vi "Insert_Event_Log(Error_glue).vi"(8 "data":string="790", 9 "message":string="B", 10 "id":string="NG", 11 "DBlink":string="Driver={ODBC Driver 17 for SQL Server};Server=localhost\\SQLEXPRESS;Database=ZDX201;UID=labview;PWD=Dsa@54137926") -> ()   [LabVIEW 2019]
uses:
  <vilib>/addons/database/Connection.llb/DB Tools Open Connec (String).vi
  <vilib>/addons/database/NI_Database_API.lvlib
panel:
  in  "error in (no error)":errorcluster
  out "error out":errorcluster
  in  "Insert value":T1={"id"="790", "classify"=1, "message"="NG", "data"="B"}
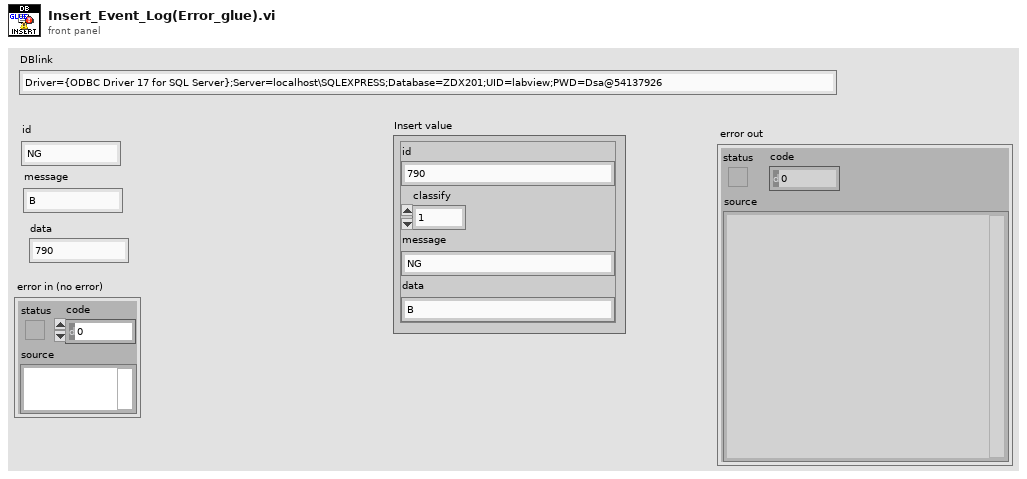
[diagram p1: front panel]
types:
  T1 = cluster{"id":string, "classify":i16, "message":string, "data":string}
  T2 = typedef "NI_Database_API.lvlib/Conn ObjectReference.ctl" = refnum<k1>
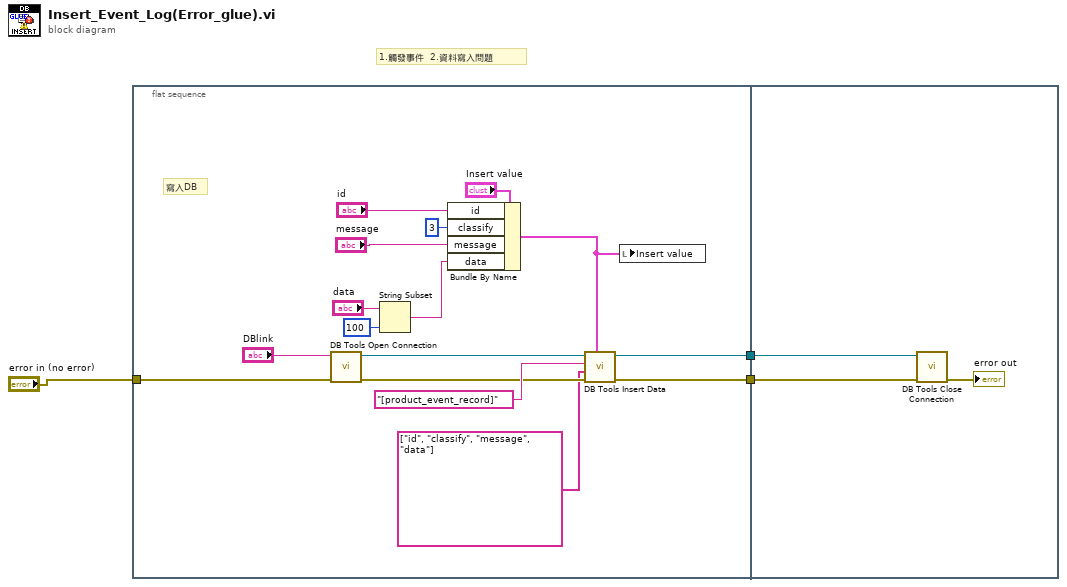
[diagram p0: block diagram]
diagram:
  # "1.觸發事件  2.資料寫入問題"
  n1 = flat-sequence {
    tunnel: [w18] -> w3
    tunnel: [w19] -> w2
    tunnel: "error in (no error)" -> [w10]
    tunnel: w3 -> [w20]
    tunnel: w2 -> [w21]
    frame #0 {
      # "寫入DB"
      n2 = call-poly <vilib>:"DB Tools Open Connection.vi"("error in (no error)"=w10, "connection information"="DBlink") -> ("error out"=w16:errorcluster, "connection reference"=w15:T2)  [unwired: 6 in]
      n3 = String Subset(string="data", length (rest)=100 ("length (rest)")) -> (substring=w4:string)  [unwired: 1 in]
      n4 = Bundle By Name(cluster="Insert value", "id"="id", "classify"=i16 3, "message"="message", "data"=w4) -> (w12:T1)
      n5 = call <vilib>:"DB Tools Insert Data.vi"("data"=w12, "error in (no error)"=w16, "columns"=string[] ["id", "classify", "message", "data"], "table"="[product_event_record]", "connection reference"=w15) -> ("error out"=w18:errorcluster, "connection reference out"=w19:T2)  [unwired: 5 in]
      n6 = local write "Insert value"(w12) -> ()
    }
    frame #1 {
      n7 = call <vilib>:"DB Tools Close Connection.vi"("error in (no error)"=w20, "connection reference"=w21) -> ("error out"=→"error out":errorcluster)  [unwired: 5 in]
    }
  }
